vi "Generador_Senal_conv_B.vi"(8 "Vertical Fill Slide":dbl(slide) scale=-4.0..4.0, 9 "df":dbl, 10 "to":dbl, 11 "tf":dbl) -> (1 "X2":dbl[](array[numeric]))   [LabVIEW 2017]
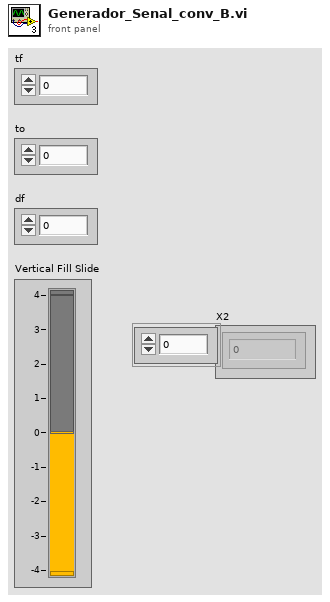
[diagram p1: front panel]
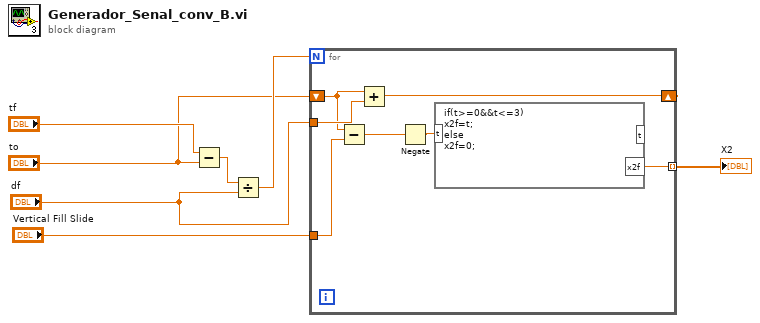
[diagram p0: block diagram]
diagram:
  n1 = Subtract(x="tf", y="to") -> (x-y=w3:dbl)
  n2 = Divide(x=w3, y="df") -> (x/y=w4:dbl)
  n3 = for {
    N: w4 -> [_]
    shift-right: [w14] -> _
    shift-left: "to" -> [w10]
    tunnel: "df" -> [w13]
    tunnel: [w12] -> w7 mode=indexing
    tunnel: "Vertical Fill Slide" -> [w11]
    n4 = Subtract(x=w10, y=w11) -> (x-y=w9:dbl)
    n5 = Add(x=w10, y=w13) -> (x+y=w14:dbl)
    n6 = Negate(x=w9) -> (-x=w8:dbl)
    n7 = formula code="if(t>=0&&t<=3)\nx2f=t;\nelse\nx2f=0;"("t"=w8) -> ("x2f"=w12:dbl)  [unwired: 1 out]
  }
  "X2" <- w7
